vi "SetParam.vi"(8 "error in (no error)":errorcluster caption="entrée d'erreur (pas d'erreur)", 10 "paired_distances":cluster{"metric":string}={"metric"="euclidean"}, 11 "Paired_distances.lvclass":refnum<class "Paired_distances.lvclass">) -> (0 "error out":errorcluster caption="sortie d'erreur", 3 "Paired_distances.lvclass":refnum<class "Paired_distances.lvclass">)   [LabVIEW 2020, in "Paired_distances.lvclass"]
doc: "Set Parameters"
uses:
  Paired_distances.lvclass
  Paired_distances.lvclass/Paired_distances.ctl
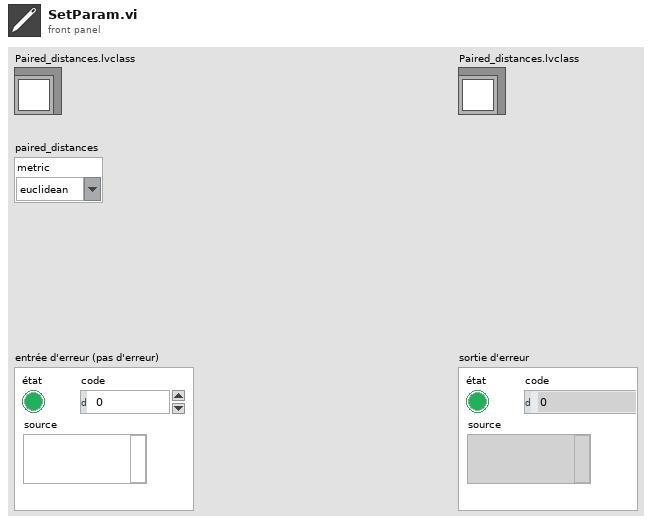
[diagram p1: front panel]
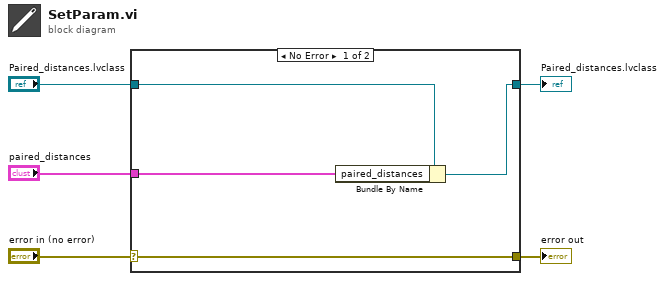
[diagram p0: block diagram]
diagram:
  n1 = case shown="No Error" "error in (no error)" {
    selector: "error in (no error)" -> [w9 w10]
    tunnel: [w9 w10] -> w4
    tunnel: [w7 w11] -> w2
    tunnel: "Paired_distances.lvclass" -> [w8 w11]
    tunnel: "paired_distances" -> [w6 _]
    frame No Error {
      n2 = Bundle By Name(cluster=w8, "paired_distances"=w6) -> (w7:refnum<class "Paired_distances.lvclass">)
    }
    frame Error {
    }
  }
  "error out" <- w4
  "Paired_distances.lvclass" <- w2
